vi "TestStimulate.vi"() -> ()   [LabVIEW 2015]
panel:
  out "Waveform Graph":dynamicdata(graph)
  in  "Size":dbl
  in  "stop":bool
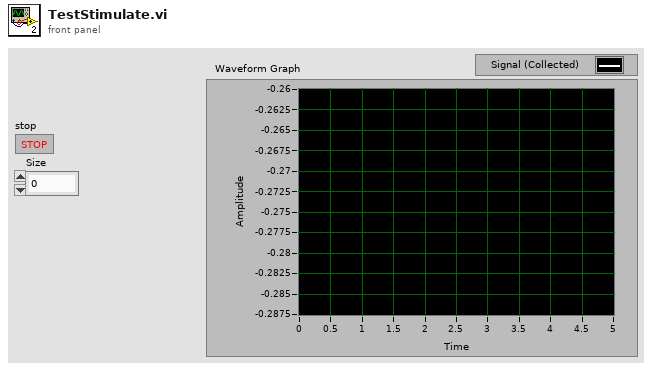
[diagram p1: front panel]
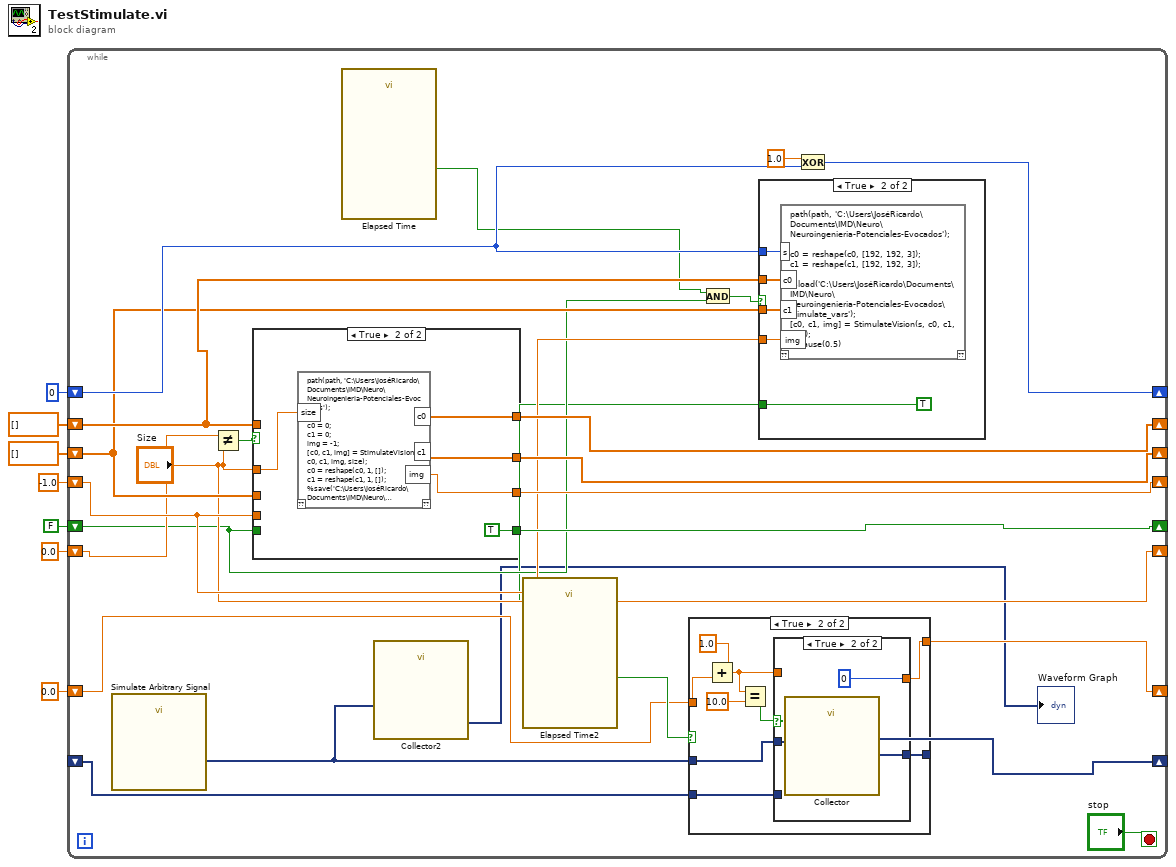
[diagram p0: block diagram]
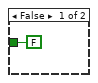
[diagram p4: hidden frame]
diagram:
  n1 = while {
    shift-right: [w29] -> _
    shift-left: 0 -> [w30]
    shift-right: [w27] -> _
    shift-left: FALSE -> [w18]
    shift-right: [w26] -> _
    shift-left: dbl[] [] -> [w23]
    shift-right: [w25] -> _
    shift-left: dbl[] [] -> [w22]
    shift-right: [w24] -> _
    shift-left: -1.0 -> [w21]
    shift-right: ["Size"] -> _
    shift-left: 0.0 ("Size") -> [w20]
    shift-right: [w12] -> _
    shift-left: 0.0 -> [w13]
    shift-right: [w10] -> _
    shift-left: _ -> [w11]
    stop <- "stop" stop-if-true
    n2 = call "Simulate Arbitrary Signal"() -> ("Signal"=w9:dynamicdata)  [unwired: 9 in, 2 out]
    n3 = Not Equal?(x=w20, y="Size") -> (x != y?=w28:bool)
    n4 = case shown="True" w28 {
      tunnel: [w58 TRUE] -> w27
      tunnel: "Size" -> [_ w62]
      tunnel: w18 -> [w58 _]
      tunnel: [w55 w61] -> w26
      tunnel: [w57 w60] -> w25
      tunnel: [w56 w59] -> w24
      tunnel: w23 -> [w55 _]
      tunnel: w22 -> [w57 _]
      tunnel: w21 -> [w56 _]
      frame False {
      }
      frame True {
        n5 = script code="path(path, 'C:\\Users\\JoséRicardo\\Documents\\IMD\\Neuro\\Neuroingenieria-Potenciales-Evocados');\n\nc0 = 0;\nc1 = 0;\nimg = -1;\n[c0, c1, img] = StimulateVision(s, c0, c1, img, size);\nc0 = reshape(c0, 1, []);\nc1 = reshape(c1, 1, []);\n%save('C:\\Users\\JoséRicardo\\Documents\\IMD\\Neuro\\Neuroingenieria-Potenciales-Evocados\\stimulate_vars');"("size"=w62) -> ("c0"=w61:dbl[], "c1"=w60:dbl[], "img"=w59:dbl)  [unwired: 1 in, 1 out]
      }
    }
    n6 = call "Elapsed Time"() -> ("Time has Elapsed"=w16:bool)  [unwired: 12 in, 7 out]
    n7 = call "Collector2"("Signals"=w9) -> ("Collected Signals"=→"Waveform Graph":dynamicdata)  [unwired: 9 in, 1 out]
    n8 = And(x=w16, y=w18) -> (x .and. y?=w17:bool)
    n9 = case shown="True" w17 {
      tunnel: w30 -> [_ w54]
      tunnel: w23 -> [_ w53]
      tunnel: w22 -> [_ w52]
      tunnel: w21 -> [_ w51]
      tunnel: [FALSE TRUE] -> w14
      frame False {
      }
      frame True {
        n10 = script code="path(path, 'C:\\Users\\JoséRicardo\\Documents\\IMD\\Neuro\\Neuroingenieria-Potenciales-Evocados');\n\nc0 = reshape(c0, [192, 192, 3]);\nc1 = reshape(c1, [192, 192, 3]);\n\n%load('C:\\Users\\JoséRicardo\\Documents\\IMD\\Neuro\\Neuroingenieria-Potenciales-Evocados\\stimulate_vars');\n[c0, c1, img] = StimulateVision(s, c0, c1, img);\n%pause(0.5)"("s"=w54, "c0"=w53, "c1"=w52, "img"=w51) -> ()  [unwired: 1 in, 1 out]
      }
    }
    n11 = call "Elapsed Time2"("Reset"=w14) -> ("Time has Elapsed"=w15:bool)  [unwired: 11 in, 7 out]
    n12 = case shown="True" w15 {
      tunnel: w9 -> [_ w43]
      tunnel: [w33 w42] -> w10
      tunnel: w13 -> [w34 w41]
      tunnel: [w34 w37] -> w12
      tunnel: w11 -> [w33 w35]
      frame False {
      }
      frame True {
        n13 = Add(x=1.0, y=w41) -> (x+y=w36:dbl)
        n14 = Equal?(x=w36, y=10.0) -> (x = y?=w38:bool)
        n15 = case shown="True" w38 {
          tunnel: w43 -> [_ w48]
          tunnel: [w44 w47] -> w42
          tunnel: [w45 0] -> w37
          tunnel: w36 -> [w45 _]
          tunnel: w35 -> [w44 _]
          frame False {
          }
          frame True {
            n16 = call "Collector"("Signals"=w48) -> ("Collected Signals"=w47:dynamicdata)  [unwired: 9 in, 1 out]
          }
        }
      }
    }
    n17 = Exclusive Or(1:w30, 2:1.0 ("x")) -> (0:w29:i32)
  }
